vi "Get All Tab Control Refs.vi"(10 "Page Index":i32=-1, 11 "TabControl in":refnum<vi>) -> (3 "ControlsOnPage":refnum<vi>[](array[refnum]))   [LabVIEW 2013]
doc: "Return an array of the references to all control and indicators within the top level of the specified page. If index is -1, return reference to controls on all pages."
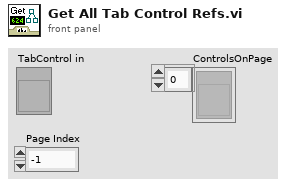
[diagram p1: front panel]
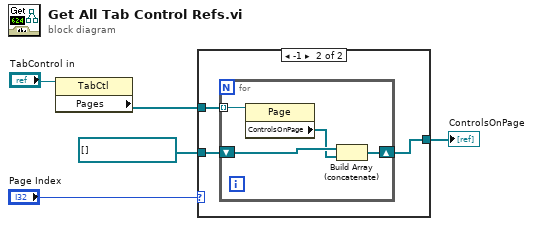
[diagram p0: block diagram]
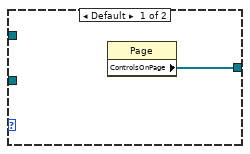
[diagram p2: hidden frame]
diagram:
  n1 = property class="TabCtl"(reference="TabControl in") -> ("Pages"=w3:refnum<vi>[])  [unwired: 1 in, 2 out]
  n2 = case shown="-1" "Page Index" {
    selector: "Page Index" -> [w6 _]
    tunnel: [w8 w9] -> w5
    tunnel: w3 -> [w7 w11]
    tunnel: refnum<vi>[] [] -> [_ w10]
    frame Default {
      n3 = property class="Page"() -> ("ControlsOnPage"=w8:refnum<vi>[])  [unwired: 2 in, 2 out]
    }
    frame -1 {
      n4 = for {
        tunnel: w11 -> [w15] mode=indexing
        shift-right: [w14] -> w9
        shift-left: w10 -> [w13]
        n5 = property class="Page"(reference=w15) -> ("ControlsOnPage"=w12:refnum<vi>[])  [unwired: 1 in, 2 out]
        n6 = Build Array (concatenate)(w13, w12) -> (w14:refnum<vi>[])
      }
    }
  }
  "ControlsOnPage" <- w5
